vi "Save-Recall Setup.vi"(8 "error in (no error)":errorcluster, 9 "Memory Location (1)":i32=1, 10 "Operation (0: Save)":i32(ring) items=["Save", "Recall"], 11 "VISA resource name":refnum<visa-resource-name>) -> (0 "error out":errorcluster, 3 "VISA resource name out":refnum<visa-resource-name>)   [LabVIEW 2014, in "Fluke 190 Series II.lvlib"]
doc: "Saves the preset setup or recalls an internally stored setup."
uses:
  Fluke 190 Series II.lvlib
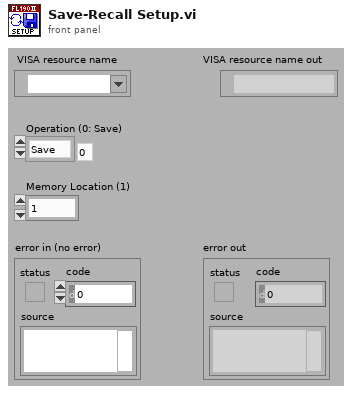
[diagram p1: front panel]
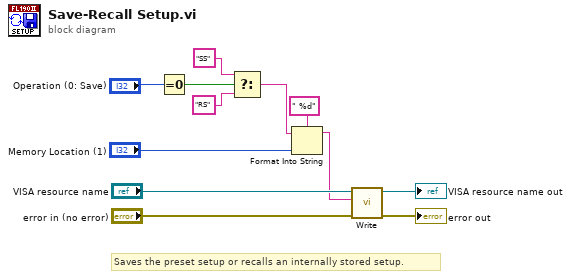
[diagram p0: block diagram]
diagram:
  # "Saves the preset setup or recalls an internally stored setup."
  n1 = Equal To 0?(x="Operation (0: Save)") -> (x = 0?=w10:bool)
  n2 = Select(t="SS", s=w10, f="RS") -> (s? t:f=w9:string)
  n3 = Format Into String(format string=" %d", initial string=w9, "Memory Location (1)") -> (resulting string=w4:string)  [unwired: 1 in, 1 out]
  n4 = call "Write.vi"("error in (no error)"="error in (no error)", "Write Buffer"=w4, "VISA resource name"="VISA resource name") -> ("error out"=→"error out":errorcluster, "VISA resource name out"=→"VISA resource name out":refnum<visa-resource-name>)  [unwired: 7 out]
